vi "Set Number And Operation On Instance.vi"(8 "error in (no error)":errorcluster, 10 "Cluster":T1, 11 "Cluster With Class":T2) -> (0 "error out":errorcluster, 3 "Cluster With Class Out":T2)   [LabVIEW 2012]
uses:
  ClassDefinitions/SimpleClassWithMethods/SimpleArithmetic.lvclass
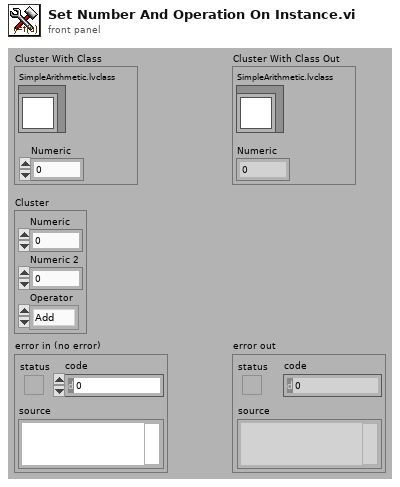
[diagram p1: front panel]
types:
  T1 = cluster{"Numeric":dbl, "Numeric 2":dbl, "Operator":enum16{"Add", "Divide", "Multiple", "Subtract"}}
  T2 = cluster{"SimpleArithmetic.lvclass":refnum<class "SimpleArithmetic.lvclass">, "Numeric":dbl}
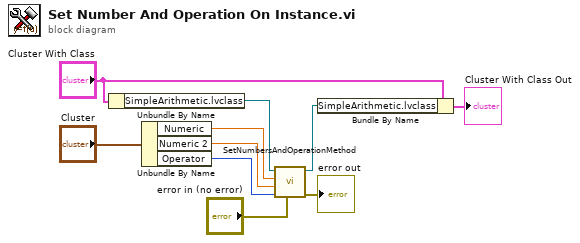
[diagram p0: block diagram]
diagram:
  n1 = Unbundle By Name("Cluster With Class") -> ("SimpleArithmetic.lvclass"=w10:refnum<class "SimpleArithmetic.lvclass">)
  n2 = Unbundle By Name("Cluster") -> ("Numeric"=w3:dbl, "Numeric 2"=w2:dbl, "Operator"=w1:enum16{"Add", "Divide", "Multiple", "Subtract"})
  n3 = call "SetNumbersAndOperationMethod.vi"("error in (no error)"="error in (no error)", "Operator"=w1, "Numeric 2"=w2, "Numeric"=w3, "SimpleArithmetic in"=w10) -> ("error out"=→"error out":errorcluster, "SimpleArithmetic out"=w7:refnum<class "SimpleArithmetic.lvclass">)  [unwired: 5 in]
  n4 = Bundle By Name(cluster="Cluster With Class", "SimpleArithmetic.lvclass"=w7) -> (→"Cluster With Class Out":T2)
